vi "BRig_dataTrial_Cue2_iTrial_Low.vi"() -> (2 "output_Cue2_iTrial_Low":i32)   [LabVIEW 2014]
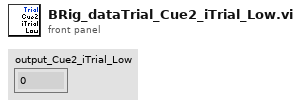
[diagram p1: front panel]
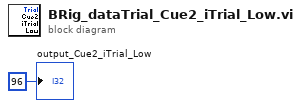
[diagram p0: block diagram]
diagram:
  "output_Cue2_iTrial_Low" <- 96 ("output_iBlock")
